vi "Publish to Local Subs.vi"(8 "error in (no error)":errorcluster, 10 "Group":refnum<class "Group.lvclass">, 11 "VolatusAPI in":refnum<class "VolatusAPI.lvclass">) -> (0 "error out":errorcluster, 3 "VolatusAPI out":refnum<class "VolatusAPI.lvclass">)   [LabVIEW 2020, in "Volatus.lvlib" / "VolatusAPI.lvclass"]
uses:
  VolatusAPI.lvclass
  lv-vecto/Vecto/Group/Group.lvclass
  VolatusAPI.lvclass/VolatusAPI.ctl
  lv-vecto/Vecto/Group/Group.lvclass/Group.ctl
  lv-vecto/Vecto/Group Config/Group Config.lvclass/Group Config.ctl
  lv-vecto/Vecto/Group DBL/Group DBL.lvclass
  lv-vecto/Vecto/Subscribed Data.ctl
  lv-vecto/Vecto/SubscribedDataHandler/SubscribedDataHandler.lvclass
  lv-vecto/Vecto/Vecto.lvlib
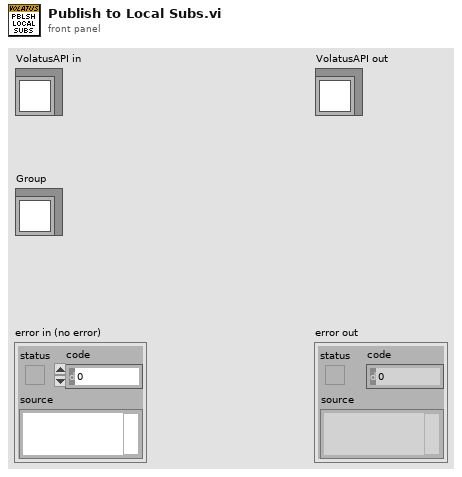
[diagram p1: front panel]
types:
  T1 = typedef "Vecto.lvlib/Subscribed Data.ctl" = cluster{"Group":string, "Timestamp":dbl, "Data":dbl[], "Received Time":dbl}
  T2 = map{string, refnum<class "SubscribedDataHandler.lvclass">[]}
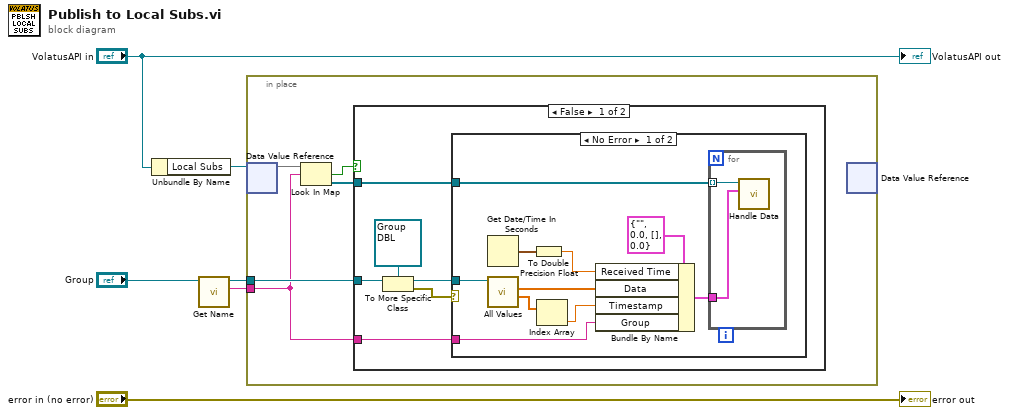
[diagram p0: block diagram]
diagram:
  n1 = Unbundle By Name("VolatusAPI in") -> ("Local Subs"=w3:refnum<data-value>)
  n2 = call "Get Name.vi"("Group in"="Group") -> ("Name"=w2:string, "Group out"=w1:refnum<class "Group.lvclass">)  [unwired: 8 in, 1 out]
  n3 = in-place {
    in-place-border: w2 -> [w7]
    in-place-border: w1 -> [w8]
    n4 = in-place-dvr #1(w3) -> (w11:T2)  [unwired: 1 out]
    n5 = Look In Map(map=w11, key=w7) -> (key not found?=w9:bool, value=w10:refnum<class "SubscribedDataHandler.lvclass">[])  [unwired: 1 in]
    n6 = case shown="False" w9 {
      tunnel: w10 -> [w17 _]
      tunnel: w8 -> [w16 _]
      tunnel: w7 -> [w12 _]
      frame False {
        n7 = To More Specific Class(target class=refnum<class "Group DBL.lvclass"> refnum ("Vecto.lvlib:Group DBL.lvclass"), reference=w16) -> (specific class reference=w13:refnum<class "Group DBL.lvclass">, error out=w14:errorcluster)  [unwired: 1 in]
        n8 = case shown="No Error" w14 {
          tunnel: w17 -> [w27 _]
          tunnel: w13 -> [w25 _]
          tunnel: w12 -> [w21 _]
          frame No Error {
            n9 = Get Date/Time In Seconds() -> (seconds since 1Jan1904=w20:timestamp)
            n10 = call "All Values.vi"("Group in"=w25) -> ("Timestamp"=w23:dbl[], "Scaled"=w24:dbl[])  [unwired: 6 in, 3 out]
            n11 = To Double Precision Float(number=w20) -> (double precision float=w19:dbl)
            n12 = Index Array(array=w23) -> (element=w22:dbl)  [unwired: 1 in]
            n13 = Bundle By Name(cluster=T1 {"Group"="", "Timestamp"=0.0, "Data"=[], "Received Time"=0.0} ("Data"), "Received Time"=w19, "Data"=w24, "Timestamp"=w22, "Group"=w21) -> (w18:T1)
            n14 = for {
              tunnel: w27 -> [w29] mode=indexing
              tunnel: w18 -> [w28]
              n15 = call-dynamic "Handle Data.vi"("Data"=w28, "SubscribedDataHandler in"=w29) -> ()  [unwired: 9 in, 1 out]
            }
          }
          frame Error {
          }
        }
      }
      frame True {
        # "Not subscribed to locally"
      }
    }
    n16 = in-place-dvr #1() -> ()  [unwired: 1 in, 2 out]
  }
  "error out" <- "error in (no error)"
  "VolatusAPI out" <- "VolatusAPI in"
